vi "Size.vi"(1 "ByteArrayTuple in":refnum<class "Bytestream.lvclass">) -> (0 "size":i32)   [LabVIEW 2020, in "NI_Bytestream.lvlib" / "Bytestream.lvclass"]
uses:
  <vilib>/Array/Bytestream/Bytestream.lvclass
  <vilib>/Array/Bytestream/Bytestream.lvclass/Bytestream.ctl
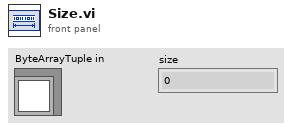
[diagram p1: front panel]
types:
  T1 = typedef "NI_Bytestream.lvlib/Bytestream.lvclass/Datum.ctl" = cluster{"array":u8[], "index":i32}
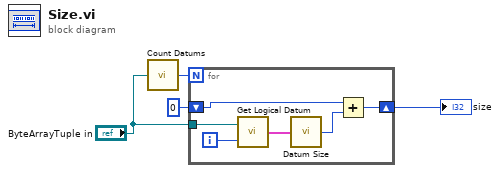
[diagram p0: block diagram]
diagram:
  n1 = call <vilib>:"Count Datums.vi"("bytestream"="ByteArrayTuple in") -> ("datums"=w2:i32)
  n2 = for {
    N: w2 -> [_]
    shift-right: [w9] -> w3
    shift-left: 0 -> [w8]
    tunnel: "ByteArrayTuple in" -> [w7]
    i -> [w6]
    n3 = call <vilib>:"Get Logical Datum.vi"("index"=w6, "bytestream"=w7) -> ("datum"=w5:T1)
    n4 = call <vilib>:"Datum Size.vi"("datum"=w5) -> ("size"=w10:i32)
    n5 = Add(x=w8, y=w10) -> (x+y=w9:i32)
  }
  "size" <- w3
